vi "Auto Drive.vi"(8 "Move":bool) -> ()   [LabVIEW 2014]
uses:
  <vilib>/Rock Robotics/WPI/RobotDrive/WPI_RobotDriveGetSetRefNum.vi
  <vilib>/Rock Robotics/WPI/RobotDrive/WPI_RobotDriveMecanumDrive_Cartesian.vi
panel:
  out "Angle":dbl
  out "Angular Rate":dbl
  in  "desired heading":dbl
  in  "multiplication control":dbl=0.1 format="%#_13g"
  out "drive strength":dbl
  in  "X":dbl format="%#_13g"
  in  "Y":dbl=-0.3 step=0.05 format="%#_13g"
  in  "Gyro Reset":bool
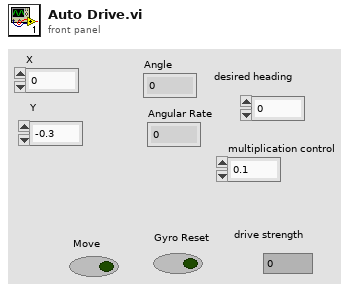
[diagram p1: front panel]
types:
  T1 = typedef "WPI_GyroDevRef.ctl" = cluster{"DevStatus":errorcluster, "Analog Module":T2, "Analog Channel":T3, "Offset":dbl, "Gain (VoltsPerDegree/Second)":dbl}
  T2 = typedef "FPGA_TypedefAnalogModule.ctl" = enum16{"Controller 1"}
  T3 = typedef "FPGA_AIChannel.ctl" = enum8{"AI 0", "AI 1", "AI 2", "AI 3", "AI MXP 0", "AI MXP 1", "AI MXP 2", "AI MXP 3", "Invalid"}
  T4 = typedef "WPI_RobotDriveDevRef.ctl" = cluster{"DevStatus":errorcluster, "Motors[]":T5[], "Square Inputs":bool, "Max Output":dbl}
  T5 = typedef "WPI_MotorControlDeviceRef.ctl" = cluster{"DeviceStatus":errorcluster, "Type":T6, "PWM":cluster{"Controller":T7, "PWM Channel":T8, "DeadBand":T9}, "CAN":cluster{"Device Number":u8, "Control Mode":T10, "Semaphore":T11, "Max Vout":dbl, "TalonSRX Control Mode":T12}, "Invert":bool, "TransformRef":T13, "InvTransformRef":T13}
  T6 = typedef "WPI_MotorControlType.ctl" = enum16{"PWM", "CAN", "CANTalonSRX"}
  T7 = typedef "FPGA_TypedefDigitalModule.ctl" = enum16{"Controller 1"}
  T8 = typedef "FPGA_DIOPWMChannel.ctl" = enum8{"PWM 0", "PWM 1", "PWM 2", "PWM 3", "PWM 4", "PWM 5", "PWM 6", "PWM 7", "PWM 8", "PWM 9", "PWM MXP 0", "PWM MXP 1", "PWM MXP 2", "PWM MXP 3", "PWM MXP 4", "PWM MXP 5", "PWM MXP 6", "PWM MXP 7", "PWM MXP 8", "PWM MXP 9", "Invalid"}
  T9 = typedef "WPI_PWMDeadband.ctl" = cluster{"Name":string, "maxPositivePwm":i32, "minPositivePwm":i32, "centerPwm":i32, "maxNegativePwm":i32, "minNegativePwm":i32, "angularRange":u16}
  T10 = typedef "WPI_CANJaguar_ControlMode.ctl" = enum8{"Percent VBus", "Current", "Speed", "Position", "Voltage"}
  T11 = typedef "Semaphore RefNum" = refnum<k1>
  T12 = typedef "WPI_CANTalonSRX_APIControlMode.ctl" = enum8{"Percent VBus", "Speed", "Position", "Slave", "Unchanged / Invalid"}
  T13 = typedef "WPI_PWMTransform_ConPane.ctl" = refnum<vi>
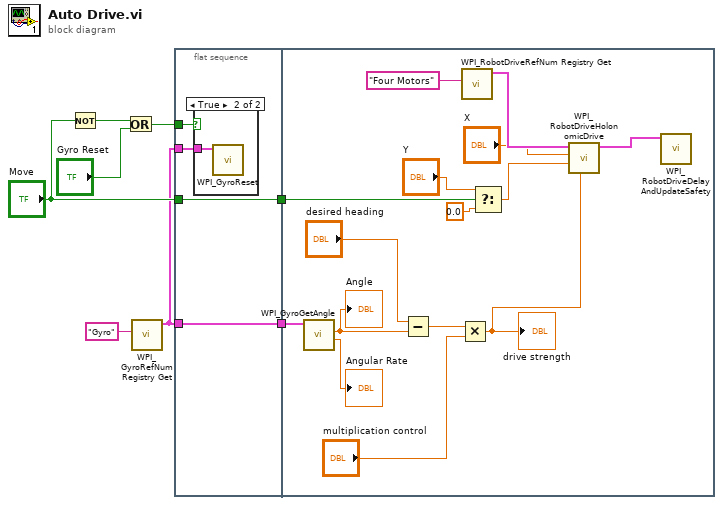
[diagram p0: block diagram]
diagram:
  n1 = Not(x="Move") -> (.not. x?=w5:bool)
  n2 = Or(x=w5, y="Gyro Reset") -> (x .or. y?=w6:bool)
  n3 = call <vilib>:"WPI_GyroRefNum Registry Get.vi"("refnum name"="Gyro") -> ("GyroDevRef"=w1:T1)  [unwired: 9 in, 1 out]
  n4 = flat-sequence {
    tunnel: w6 -> [w12]
    tunnel: w1 -> [w11]
    tunnel: "Move" -> [w10]
    tunnel: [w10] -> w3
    tunnel: [w9] -> w2
    tunnel: w1 -> [w9]
    tunnel: w3 -> [w17]
    tunnel: w2 -> [w14]
    frame #0 {
      n5 = case shown="True" w12 {
        tunnel: w11 -> [_ w13]
        frame False {
        }
        frame True {
          n6 = call <vilib>:"WPI_GyroReset.vi"("GyroDevRef"=w13) -> ()  [unwired: 9 in, 2 out]
        }
      }
    }
    frame #1 {
      n7 = call <vilib>:"WPI_GyroGetAngle.vi"("GyroDevRef"=w14) -> ("Angular Rate"=→"Angular Rate":dbl, "Angle"=w15:dbl)  [unwired: 7 in, 2 out]
      "Angle" <- w15
      n8 = Subtract(x="desired heading", y=w15) -> (x-y=w24:dbl)
      n9 = Multiply(x=w24, y="multiplication control") -> (x*y=w25:dbl)
      "drive strength" <- w25
      n10 = call <vilib>:"WPI_RobotDriveRefNum Registry Get.vi"("refnum name"="Four Motors") -> ("RobotDriveDevRef"=w20:T4)  [unwired: 1 in, 9 out]
      n11 = Select(t="Y", s=w17, f=0.0 ("t")) -> (s? t:f=w26:dbl)
      n12 = call-poly <vilib>:"WPI_RobotDriveHolonomicDrive.vi"("Rotation"=w25, "Y"=w26, "X"="X", "RobotDriveDevRef"=w20) -> ("RobotDriveDevRef"=w19:T4)  [unwired: 5 in, 2 out]
      n13 = call <vilib>:"WPI_RobotDriveDelayAndUpdateSafety.vi"("RobotDriveDevRef"=w19) -> ()  [unwired: 9 in, 2 out]
    }
  }
